vi "myRIO_BRig_RT_comm_webdav_myrioFolder.vi"() -> (2 "output_myrioFolder":string="http://172.22.11.1")   [LabVIEW 2014]
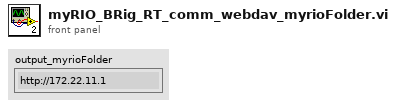
[diagram p1: front panel]
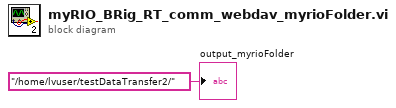
[diagram p0: block diagram]
diagram:
  "output_myrioFolder" <- "/home/lvuser/testDataTransfer2/" ("host uri prefix")
